vi "searchClusterNames.vi"(6 "Separator (\"\") 2":string="Channel 1", 9 "Command or variable":string, 10 "exact match":bool, 11 "variant (destination) 2":variant) -> (3 "element":string, 4 "Array 2":bool[](array[boolean]))   [LabVIEW 2011]
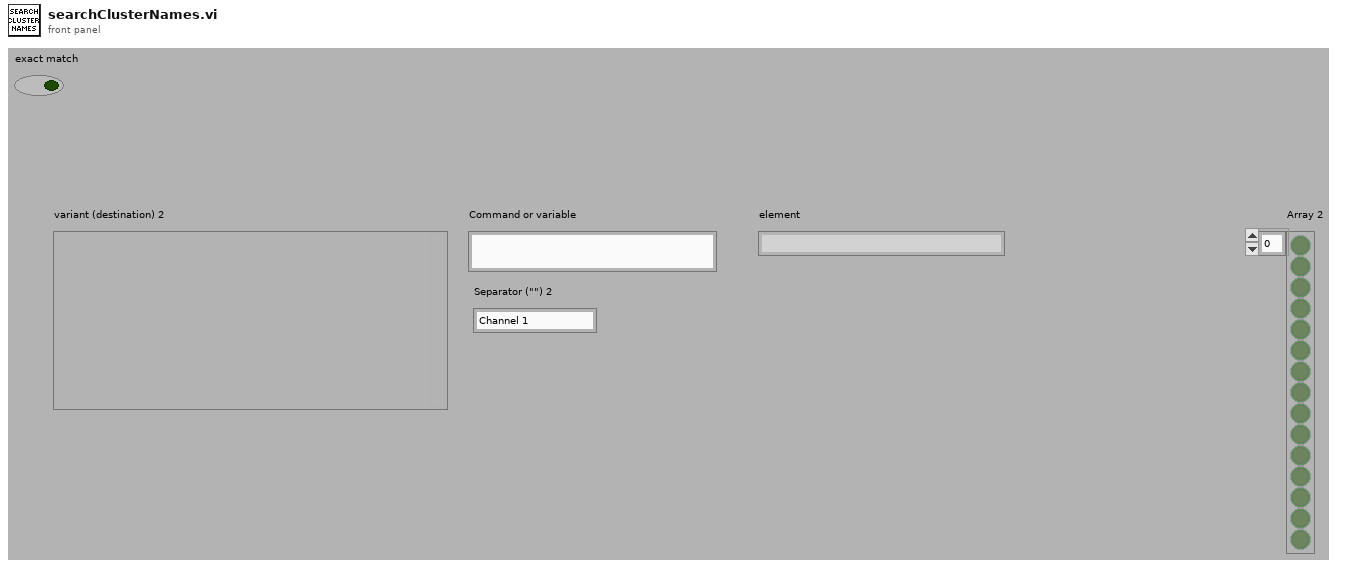
[diagram p1: front panel]
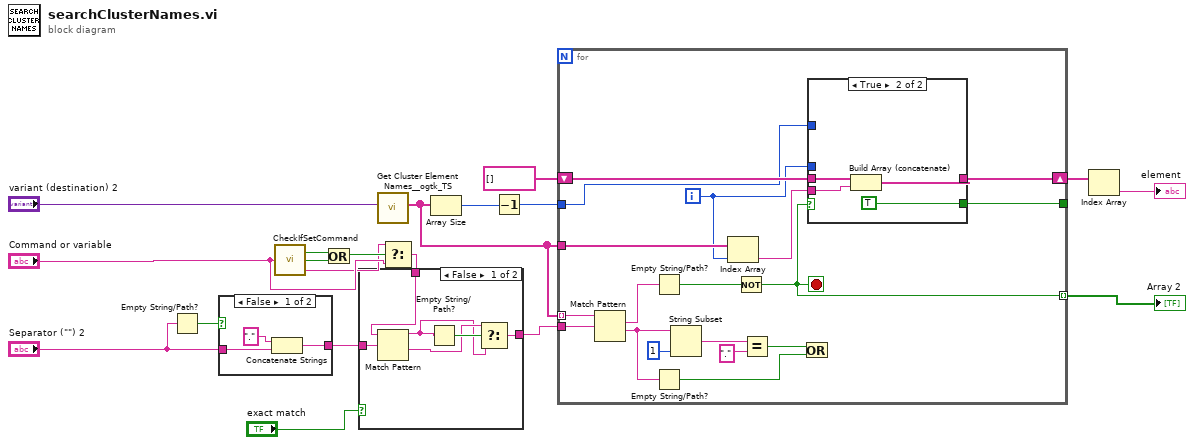
[diagram p0: block diagram]
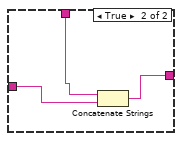
[diagram p2: hidden frame]
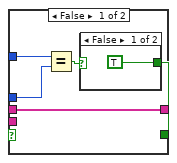
[diagram p4: hidden frame]
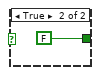
[diagram p5: hidden frame]
diagram:
  n1 = Empty String/Path?(string/path="Separator (\"\") 2") -> (empty?=w14:bool)
  n2 = case shown="False" w14 {
    tunnel: "Separator (\"\") 2" -> [w21 w23]
    tunnel: [w20 w23] -> w15
    frame False {
      n3 = Concatenate Strings("." ("string"), w21) -> (w20:string)
    }
    frame True {
    }
  }
  n4 = call "CheckIfSetCommand.vi"("Command"="Command or variable") -> ("setCommand?"=w7:bool, "getCommand?"=w6:bool, "variable"=w3:string)
  n5 = Or(x=w7, y=w6) -> (x .or. y?=w5:bool)
  n6 = call "Get Cluster Element Names__ogtk_TS.vi"("Variant"="variant (destination) 2") -> ("Names (Array)"=w12:string[])  [unwired: 9 in, 1 out]
  n7 = Select(t=w3, s=w5, f="Command or variable") -> (s? t:f=w2:string)
  n8 = case shown="False" "exact match" {
    tunnel: [w24 w30] -> w16
    tunnel: w15 -> [w28 w31]
    tunnel: w2 -> [w27 w32]
    frame False {
      n9 = Match Pattern(string=w27, regular expression=w28) -> (before substring=w25:string, after substring=w26:string)  [unwired: 1 in, 2 out]
      n10 = Empty String/Path?(string/path=w25) -> (empty?=w29:bool)
      n11 = Select(t=w26, s=w29, f=w25) -> (s? t:f=w24:string)
    }
    frame True {
      n12 = Concatenate Strings(w32, w31) -> (w30:string)
    }
  }
  n13 = Array Size(array=w12) -> (size(s)=w8:i32)
  n14 = Decrement(x=w8) -> (x-1=w9:i32)
  n15 = for {
    tunnel: w12 -> [w50] mode=indexing
    tunnel: w16 -> [w49]
    tunnel: w12 -> [w47]
    shift-right: [w45] -> w17
    shift-left: string[] [] ("Element Names") -> [w44]
    tunnel: w9 -> [w36]
    tunnel: [w34] -> _
    tunnel: [w33] -> w10 mode=indexing
    i -> [w35]
    stop <- w33 stop-if-true
    n16 = Match Pattern(string=w50, regular expression=w49) -> (match substring=w48:string, after substring=w39:string)  [unwired: 1 in, 2 out]
    n17 = Empty String/Path?(string/path=w48) -> (empty?=w43:bool)
    n18 = Empty String/Path?(string/path=w39) -> (empty?=w38:bool)
    n19 = String Subset(string=w39, length (rest)=1 ("length (rest)")) -> (substring=w41:string)  [unwired: 1 in]
    n20 = Index Array(array=w47, index=w35) -> (element=w46:string)
    n21 = Not(x=w43) -> (.not. x?=w33:bool)
    n22 = Equal?(x=w41, y=".") -> (x = y?=w37:bool)
    n23 = Or(x=w37, y=w38) -> ()  [unwired: 1 out]
    n24 = case shown="True" w33 {
      tunnel: w46 -> [_ w61]
      tunnel: [w55 w60] -> w45
      tunnel: w44 -> [w55 w59]
      tunnel: w36 -> [w54 _]
      tunnel: w35 -> [w53 _]
      tunnel: [w51 TRUE] -> w34
      frame False {
        n25 = Equal?(x=w54, y=w53) -> (x = y?=w52:bool)
        n26 = case shown="False" w52 {
          tunnel: [TRUE FALSE] -> w51
          frame False {
          }
          frame True {
          }
        }
      }
      frame True {
        n27 = Build Array (concatenate)(w59, w61) -> (w60:string[])
      }
    }
  }
  "Array 2" <- w10
  n28 = Index Array(array=w17) -> (element=→"element":string)  [unwired: 1 in]
